vi "Read Setpoint.vi"(8 "error in (no error)":errorcluster, 11 "Bioreactor in":refnum<class "Bioreactor.lvclass">) -> (0 "error out":errorcluster, 3 "Bioreactor out":refnum<class "Bioreactor.lvclass">)   [LabVIEW 2013, in "Bioreactor.lvlib" / "Bioreactor.lvclass"]
uses:
  Bioreactor.lvclass
  Bioreactor.lvclass/Bioreactor.ctl
  Read Loop Name.vi
  Read Address.vi
  Read VISA resource name.vi
  PluginInterface/PluginInterface.lvlibp/PluginInterfaceClass/Read DVR.vi
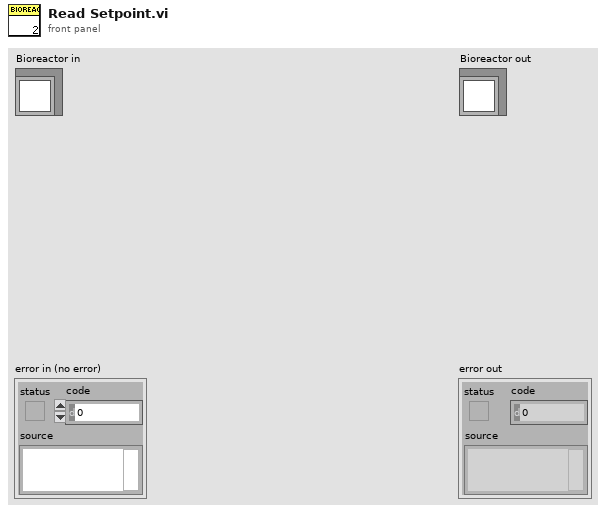
[diagram p1: front panel]
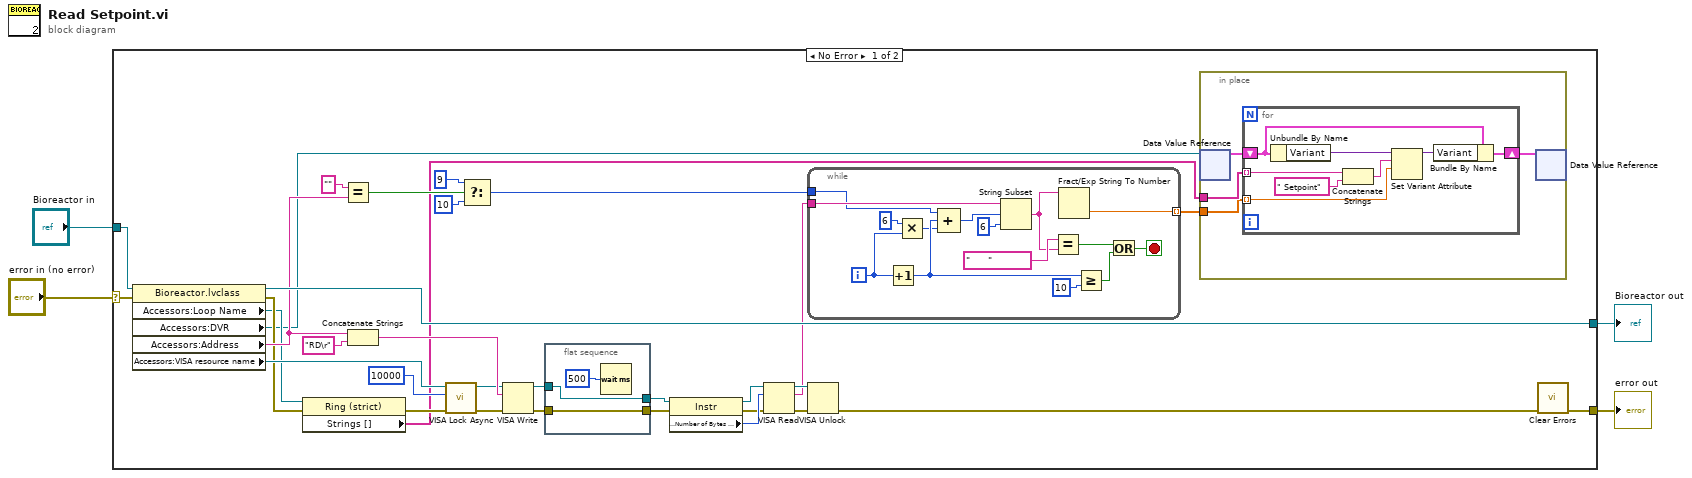
[diagram p0: block diagram]
diagram:
  n1 = case shown="No Error" "error in (no error)" {
    selector: "error in (no error)" -> [w28 w69]
    tunnel: [w6 w69] -> w1
    tunnel: [w20 w68] -> w2
    tunnel: "Bioreactor in" -> [w27 w68]
    frame No Error {
      n2 = property class="Bioreactor.lvclass"(reference=w27, error in=w28) -> (reference out=w20:refnum<class "Bioreactor.lvclass">, error out=w12:errorcluster, "Accessors:Loop Name"=w10:refnum<vi>, "Accessors:DVR"=w9:refnum<data-value>, "Accessors:Address"=w13:string, "Accessors:VISA resource name"=w21:refnum<visa-resource-name>)
      n3 = property class="Ring (strict)"(reference=w10, error in=w12) -> (error out=w11:errorcluster, "Strings []"=w8:string[])  [unwired: 1 out]
      n4 = Equal?(x="", y=w13) -> (x = y?=w18:bool)
      n5 = Concatenate Strings(w13, "RD\r") -> (w29:string)
      n6 = call <vilib>:"VISA Lock Async.vi"("error in (no error)"=w11, "timeout (0)"=u32 10000, "VISA resource name"=w21) -> ("error out"=w26:errorcluster, "VISA resource name out"=w25:refnum<visa-resource-name>)  [unwired: 6 in, 1 out]
      n7 = Select(t=9, s=w18, f=10) -> (s? t:f=w14:i32)
      n8 = VISA Write(VISA resource name=w25, write buffer=w29, error in (no error)=w26) -> (VISA resource name out=w34:refnum<visa-resource-name>, error out=w32:errorcluster)  [unwired: 1 out]
      n9 = flat-sequence {
        tunnel: [w67] -> w33
        tunnel: w34 -> [w67]
        tunnel: [w66] -> w31
        tunnel: w32 -> [w66]
        frame #0 {
          n10 = Wait (ms)(milliseconds to wait=500 ("y")) -> ()  [unwired: 1 out]
        }
      }
      n11 = property class="Instr"(reference=w33, error in=w31) -> (reference out=w35:refnum<visa-resource-name>, error out=w36:errorcluster, "Serial Settings:Number of Bytes at Serial Port"=w37:u32)
      n12 = VISA Read(VISA resource name=w35, byte count=w37, error in (no error)=w36) -> (VISA resource name out=w22:refnum<visa-resource-name>, read buffer=w19:string, error out=w23:errorcluster)  [unwired: 1 out]
      n13 = while {
        tunnel: w19 -> [w64]
        tunnel: w14 -> [w63]
        tunnel: [w50] -> w7 mode=indexing
        i -> [w54]
        stop <- w57 stop-if-true
        n14 = Increment(x=w54) -> (x+1=w60:i32)
        n15 = Multiply(x=6, y=w54) -> (x*y=w53:i32)
        n16 = Compound Arithmetic op=ADD(w63, w60, w53) -> (w62:i32)
        n17 = String Subset(string=w64, offset (0)=w62, length (rest)=6) -> (substring=w51:string)
        n18 = Equal?(x="      " ("y"), y=w51) -> (x = y?=w61:bool)
        n19 = Fract/Exp String To Number(string=w51) -> (number=w50:dbl)  [unwired: 3 in, 1 out]
        n20 = Greater Or Equal?(x=w60, y=10) -> (x >= y?=w58:bool)
        n21 = Or(x=w61, y=w58) -> (x .or. y?=w57:bool)
      }
      n22 = VISA Unlock(8:w23, 11:w22) -> (0:w5:errorcluster)  [unwired: 1 out]
      n23 = in-place {
        in-place-border: w8 -> [w41]
        in-place-border: w7 -> [w38]
        n24 = in-place-dvr #1(w9) -> (w40:cluster{"Array":string[], "Variant":variant})  [unwired: 1 out]
        n25 = for {
          tunnel: w41 -> [w49] mode=indexing
          tunnel: w38 -> [w46] mode=indexing
          shift-right: [w42] -> w39
          shift-left: w40 -> [w45]
          n26 = Unbundle By Name(w45) -> ("Variant"=w44:variant)
          n27 = Concatenate Strings(w49, " Setpoint" ("string")) -> (w47:string)
          n28 = Set Variant Attribute(Variant=w44, name=w47, value=w46) -> (Variant out=w43:variant)  [unwired: 1 in, 2 out]
          n29 = Bundle By Name(cluster=w45, "Variant"=w43) -> (w42:cluster{"Array":string[], "Variant":variant})
        }
        n30 = in-place-dvr #1(w39) -> ()  [unwired: 2 out]
      }
      n31 = call <vilib>:"Clear Errors.vi"("error in (no error)"=w5) -> ("error out"=w6:errorcluster)  [unwired: 6 in]
    }
    frame Error {
    }
  }
  "error out" <- w1
  "Bioreactor out" <- w2
